vi "Latch.vi"(1 "Edge":bool=TRUE, 2 "In":bool) -> (0 "Out":bool)   [LabVIEW 2012]
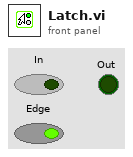
[diagram p1: front panel]
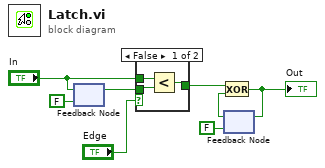
[diagram p0: block diagram]
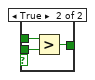
[diagram p2: hidden frame]
diagram:
  n1 = feedback #1(FALSE ("In")) -> (w8:bool)
  n2 = feedback-in #1("In") -> ()
  n3 = case shown="False" "Edge" {
    tunnel: w8 -> [w9 w14]
    tunnel: "In" -> [w10 w13]
    tunnel: [w11 w12] -> w5
    frame False {
      n4 = Less?(x=w10, y=w9) -> (x < y?=w11:bool)
    }
    frame True {
      n5 = Greater?(x=w13, y=w14) -> (0:w12:bool)
    }
  }
  n6 = feedback #2(FALSE) -> (w3:bool)
  n7 = Exclusive Or(1:w3, 2:w5) -> (0:w4:bool)
  "Out" <- w4
  n8 = feedback-in #2(w4) -> ()
